vi "start_all_backup.vi"(8 "error in (no error)":errorcluster, 11 "Handle In":i32) -> (0 "error out":errorcluster, 3 "Handle Out":i32)   [LabVIEW 2025]
uses:
  LabJackEKG.lvlib
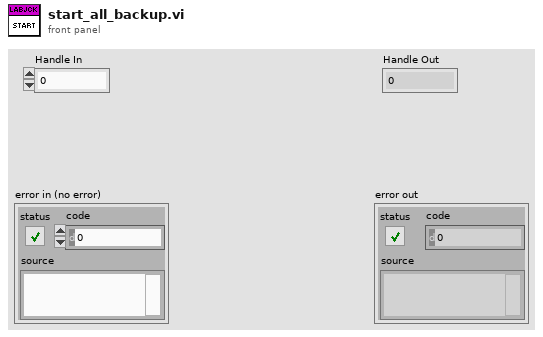
[diagram p1: front panel]
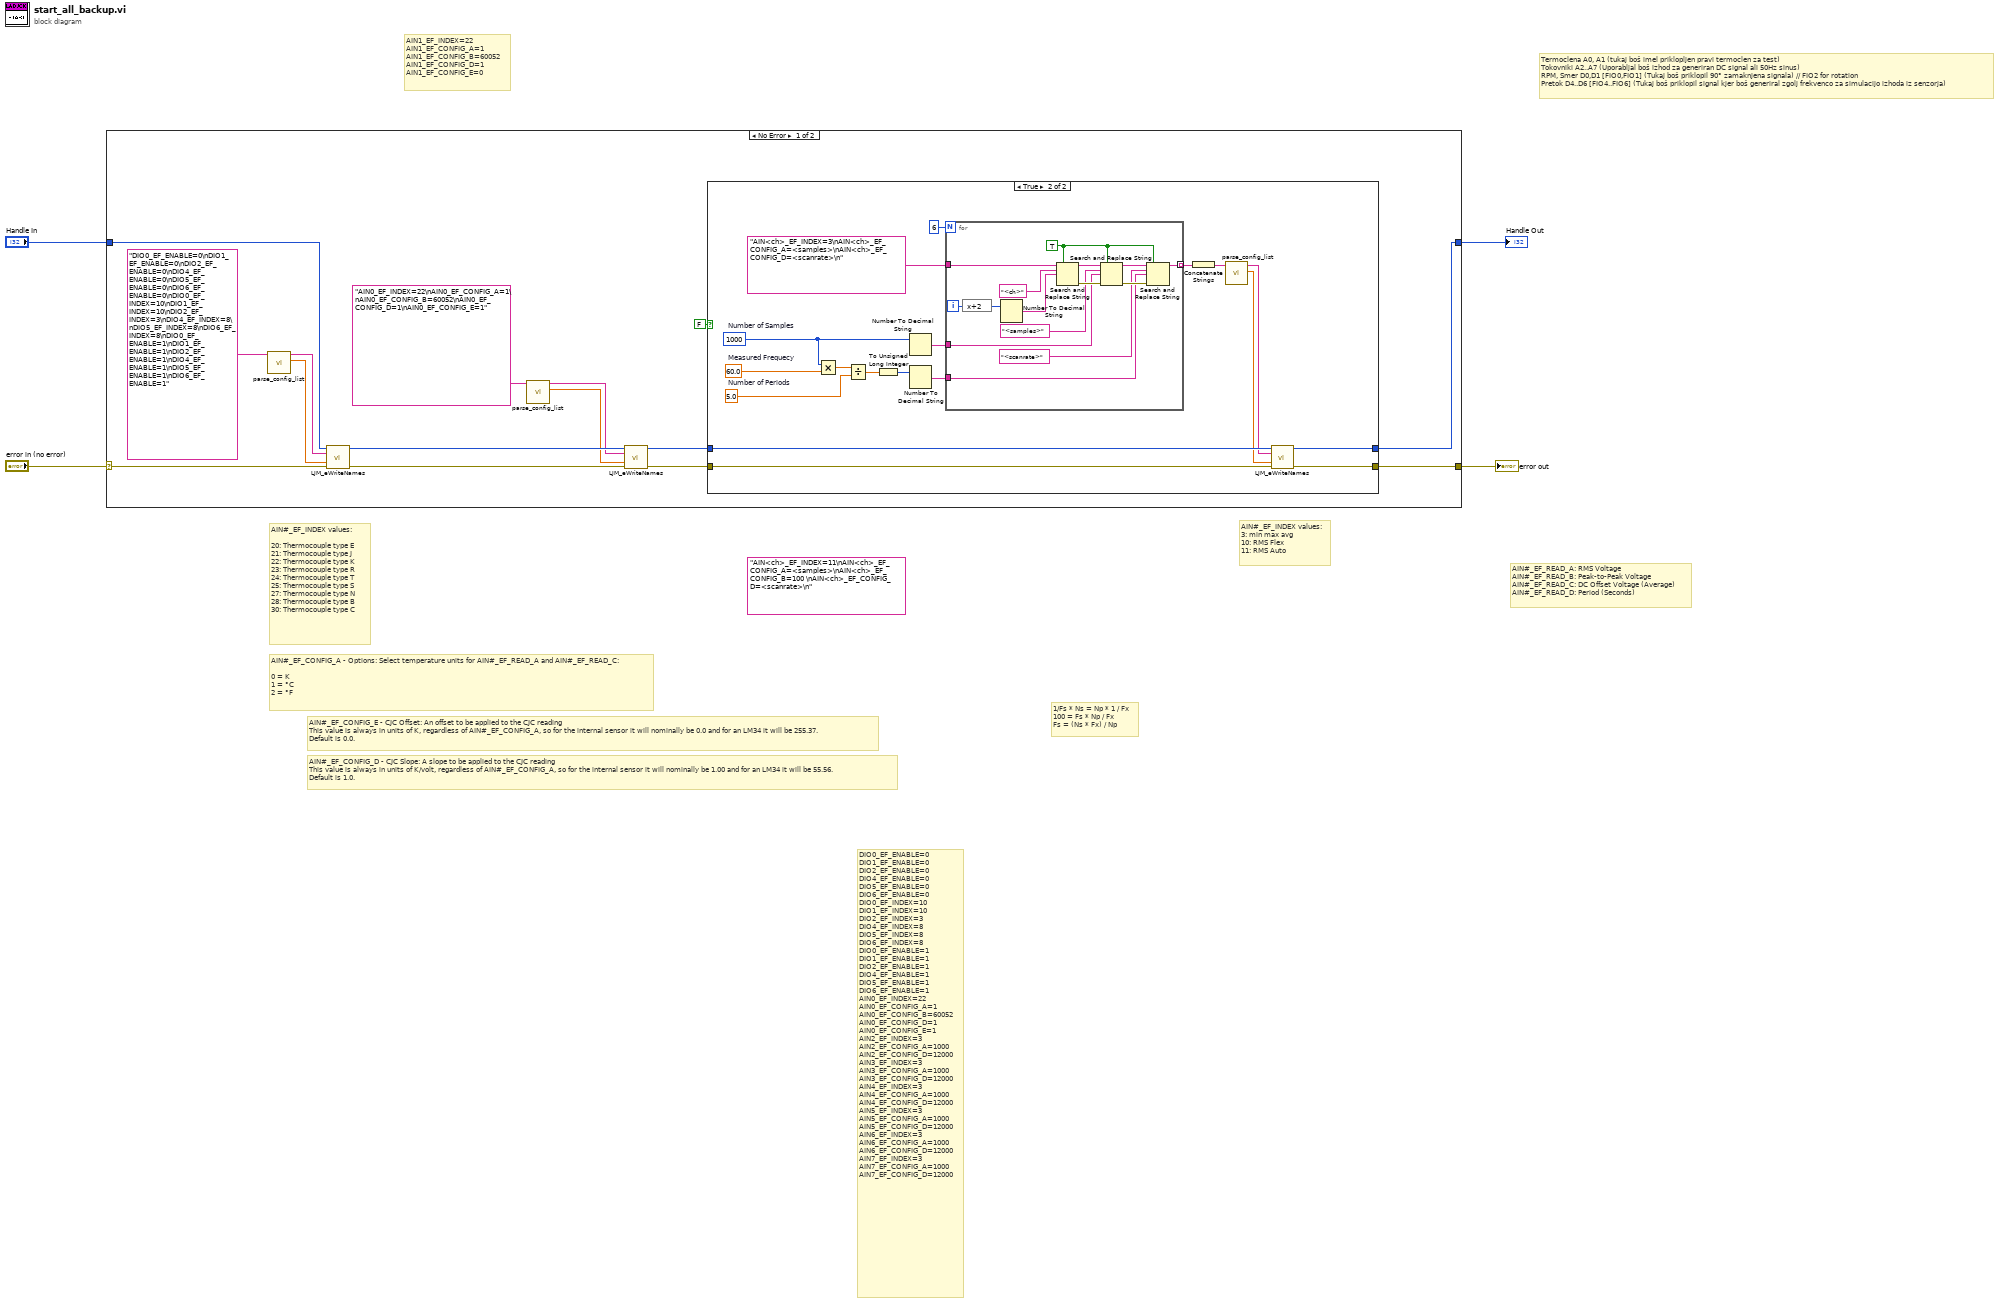
[diagram p0: block diagram]
diagram:
  (unwired) "AIN<ch>_EF_INDEX=11\nAIN<ch>_EF_CONFIG_A=<samples>\nAIN<ch>_EF_CONFIG_B=100 \nAIN<ch>_EF_CONFIG_D=<scanrate>\n"
  # "DIO0_EF_ENABLE=0\nDIO1_EF_ENABLE=0\nDIO2_EF_ENABLE=0\nDIO4_EF_ENABLE=0\nDIO5_EF_ENABLE=0\nDIO6_EF_ENABLE=0\nDIO0_EF_INDEX=10\nDIO1_EF_INDEX=10\nDIO2_EF_INDEX=3\nDIO4_EF_INDEX=8\nDIO5_EF_INDEX=8\nDIO6_EF_INDEX=8\nDIO0_EF_ENABLE=1\nDIO1_EF_ENABLE=1\nDIO2_EF_ENABLE=1\nDIO4_EF_ENABLE=1\nDIO5_EF_ENABLE=1\nDIO6_EF_ENABLE=1\nAIN0_EF_INDEX=22\nAIN0_EF_CONFIG_A=1\nAIN0_EF_CONFIG_B=60052\nAIN0_EF_CONFIG_D=1\nAIN0_EF_CONFIG_E=1\nAIN2_EF_INDEX=3\nAIN2_EF_CONFIG_A=1000\nAIN2_EF_CONFIG_D=12000\nAIN3_EF_INDEX=3\nAIN3_EF_CONFIG_A=1000\nAIN3_EF_CONFIG_D=12000\nAIN4_EF_INDEX=3\nAIN4_EF_CONFIG_A=1000\nAIN4_EF_CONFIG_D=12000\nAIN5_EF_INDEX=3\nAIN5_EF_CONFIG_A=1000\nAIN5_EF_CONFIG_D=12000\nAIN6_EF_INDEX=3\nAIN6_EF_CONFIG_A=1000\nAIN6_EF_CONFIG_D=12000\nAIN7_EF_INDEX=3\nAIN7_EF_CONFIG_A=1000\nAIN7_EF_CONFIG_D=12000"
  # "1/Fs * Ns = Np * 1 / Fx\n100 = Fs * Np / Fx\nFs = (Ns * Fx) / Np"
  # "AIN1_EF_INDEX=22\nAIN1_EF_CONFIG_A=1\nAIN1_EF_CONFIG_B=60052\nAIN1_EF_CONFIG_D=1\nAIN1_EF_CONFIG_E=0"
  # "AIN#_EF_INDEX values:\n3: min max avg\n10: RMS Flex\n11: RMS Auto"
  # "AIN#_EF_READ_A: RMS Voltage\nAIN#_EF_READ_B: Peak-to-Peak Voltage\nAIN#_EF_READ_C: DC Offset Voltage (Average)\nAIN#_EF_READ_D: Period (Seconds)"
  # "AIN#_EF_CONFIG_E - CJC Offset: An offset to be applied to the CJC reading\nThis value is always in units of K, regardless of AIN#_EF_CONFIG_A, so for the internal sensor it will nominally be 0.0 and for an LM34 it will be 255.37.\nDefault is 0.0."
  # "AIN#_EF_CONFIG_D - CJC Slope: A slope to be applied to the CJC reading\nThis value is always in units of K/volt, regardless of AIN#_EF_CONFIG_A, so for the internal sensor it will nominally be 1.00 and for an LM34 it will be 55.56.\nDefault is 1.0."
  # "AIN#_EF_CONFIG_A - Options: Select temperature units for AIN#_EF_READ_A and AIN#_EF_READ_C:\n\n0 = K\n1 = °C\n2 = °F"
  # "AIN#_EF_INDEX values:\n\n20: Thermocouple type E\n21: Thermocouple type J\n22: Thermocouple type K\n23: Thermocouple type R\n24: Thermocouple type T \n25: Thermocouple type S\n27: Thermocouple type N\n28: Thermocouple type B\n30: Thermocouple type C"
  # "Termoclena A0, A1 (tukaj boš imel priklopljen pravi termoclen za test)\nTokovniki A2..A7 (Uporabljal boš izhod za generiran DC signal ali 50Hz sinus)\nRPM, Smer D0,D1 [FIO0,FIO1] (Tukaj boš priklopil 90° zamaknjena signala) // FIO2 for rotation\nPretok D4..D6 [FIO4..FIO6] (Tukaj boš priklopil signal kjer boš generiral zgolj frekvenco za simulacijo izhoda iz senzorja)"
  n1 = case shown="No Error" "error in (no error)" {
    selector: "error in (no error)" -> [w18 w56]
    tunnel: [w8 w55] -> w4
    tunnel: "Handle In" -> [w17 w55]
    tunnel: [w6 w56] -> w1
    frame No Error {
      n2 = call "parse_config_list.vi"("String"="DIO0_EF_ENABLE=0\nDIO1_EF_ENABLE=0\nDIO2_EF_ENABLE=0\nDIO4_EF_ENABLE=0\nDIO5_EF_ENABLE=0\nDIO6_EF_ENABLE=0\nDIO0_EF_INDEX=10\nDIO1_EF_INDEX=10\nDIO2_EF_INDEX=3\nDIO4_EF_INDEX=8\nDIO5_EF_INDEX=8\nDIO6_EF_INDEX=8\nDIO0_EF_ENABLE=1\nDIO1_EF_ENABLE=1\nDIO2_EF_ENABLE=1\nDIO4_EF_ENABLE=1\nDIO5_EF_ENABLE=1\nDIO6_EF_ENABLE=1") -> ("Values"=w16:dbl[], "Names"=w15:string[])  [unwired: 9 in]
      n3 = call <vilib>:"LJM_eWriteNames.vi"("Handle In"=w17, "aNames"=w15, "aValuesIn"=w16, "error in"=w18) -> ("Handle Out"=w14:i32, "error out"=w13:errorcluster)  [unwired: 9 in, 1 out]
      n4 = call "parse_config_list.vi"("String"="AIN0_EF_INDEX=22\nAIN0_EF_CONFIG_A=1\nAIN0_EF_CONFIG_B=60052\nAIN0_EF_CONFIG_D=1\nAIN0_EF_CONFIG_E=1") -> ("Values"=w11:dbl[], "Names"=w10:string[])  [unwired: 9 in]
      n5 = call <vilib>:"LJM_eWriteNames.vi"("Handle In"=w14, "aNames"=w10, "aValuesIn"=w11, "error in"=w13) -> ("Handle Out"=w9:i32, "error out"=w7:errorcluster)  [unwired: 9 in, 1 out]
      n6 = case shown="True" FALSE {
        tunnel: w9 -> [w21 w39]
        tunnel: [w21 w38] -> w8
        tunnel: w7 -> [w20 w37]
        tunnel: [w20 w36] -> w6
        frame False {
        }
        frame True {
          w24 = 5.0  # Number of Periods
          w26 = 60.0  # Measured Frequecy
          w27 = 1000  # Number of Samples
          n7 = Multiply(x=w27, y=w26) -> (x*y=w25:dbl)
          n8 = Divide(x=w25, y=w24) -> (x/y=w23:dbl)
          n9 = To Unsigned Long Integer(number=w23) -> (unsigned 32bit integer=w22:u32)
          n10 = Number To Decimal String(number=w27) -> (decimal integer string=w31:string)  [unwired: 1 in]
          n11 = Number To Decimal String(number=w22) -> (decimal integer string=w30:string)  [unwired: 1 in]
          n12 = for {
            N: 6 -> [_]
            tunnel: "AIN<ch>_EF_INDEX=3\nAIN<ch>_EF_CONFIG_A=<samples>\nAIN<ch>_EF_CONFIG_D=<scanrate>\n" -> [w54]
            tunnel: w31 -> [w41]
            tunnel: w30 -> [w40]
            tunnel: [w45] -> w32 mode=indexing
            i -> [w44]
            w52 = TRUE ("replace all? (F)")
            n13 = expression code="x+2"(w44) -> (w43:i32)
            n14 = Number To Decimal String(number=w43) -> (decimal integer string=w42:string)  [unwired: 1 in]
            n15 = Search and Replace String(replace all?=w52, input string=w54, search string="<ch>", replace string=w42) -> (result string=w49:string, error out=w51:errorcluster)  [unwired: 4 in, 2 out]
            n16 = Search and Replace String(replace all?=w52, input string=w49, search string="<samples>", replace string=w41, error in=w51) -> (result string=w48:string, error out=w53:errorcluster)  [unwired: 3 in, 2 out]
            n17 = Search and Replace String(replace all?=w52, input string=w48, search string="<scanrate>", replace string=w40, error in=w53) -> (result string=w45:string)  [unwired: 3 in, 3 out]
          }
          n18 = Concatenate Strings(w32) -> (w29:string)
          n19 = call "parse_config_list.vi"("String"=w29) -> ("Values"=w34:dbl[], "Names"=w35:string[])  [unwired: 9 in]
          n20 = call <vilib>:"LJM_eWriteNames.vi"("Handle In"=w39, "aNames"=w35, "aValuesIn"=w34, "error in"=w37) -> ("Handle Out"=w38:i32, "error out"=w36:errorcluster)  [unwired: 9 in, 1 out]
        }
      }
    }
    frame Error {
    }
  }
  "error out" <- w1
  "Handle Out" <- w4
